vi "Wait(sec) test act.vi"(0 "command text in":string[](array[string])) -> ()   [LabVIEW 2019]
panel:
  in  "wait (sec)":i32 min=0
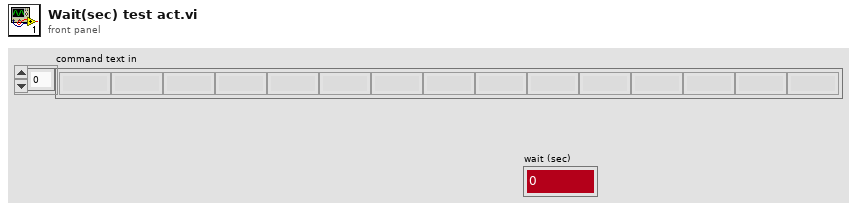
[diagram p1: front panel]
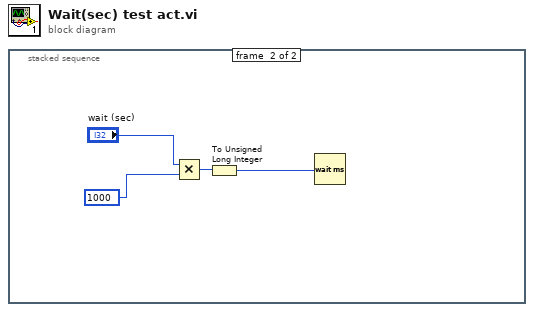
[diagram p0: block diagram]
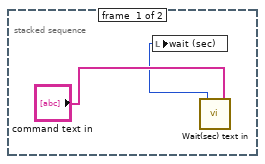
[diagram p2: hidden frame]
diagram:
  n1 = stacked-sequence {
    frame #0 {
      n2 = call "Wait(sec) text in.vi"("command text in"="command text in") -> ("extra wait (sec)"=w1:i32)
      n3 = local write "wait (sec)"(w1) -> ()
    }
    frame #1 {
      n4 = Multiply(x="wait (sec)", y=1000) -> (x*y=w4:i32)
      n5 = To Unsigned Long Integer(number=w4) -> (unsigned 32bit integer=w3:u32)
      n6 = Wait (ms)(milliseconds to wait=w3) -> ()  [unwired: 1 out]
    }
  }
